vi "FlatSequenceToJson.vi"(6 "Current Path":path, 7 "Origin Path":path, 8 "error in":errorcluster, 10 "Relative Bounds":cluster{"x":i32, "y":i32, "w":i32, "h":i32}, 11 "FlatSequence in":refnum<vi>) -> (0 "error out":errorcluster, 3 "JSON":string)   [LabVIEW 2017]
doc: "Converts a flat sequence structure into a JSON"
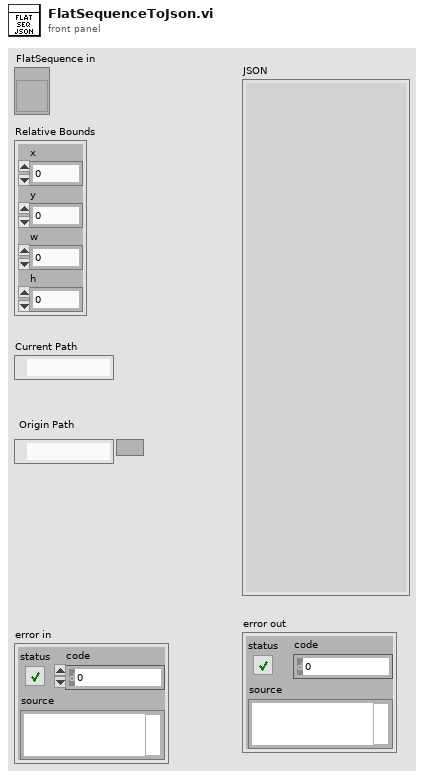
[diagram p1: front panel]
types:
  T1 = typedef "LVRectTypeDef.ctl" = cluster{"Left":i16, "Top":i16, "Right":i16, "Bottom":i16}
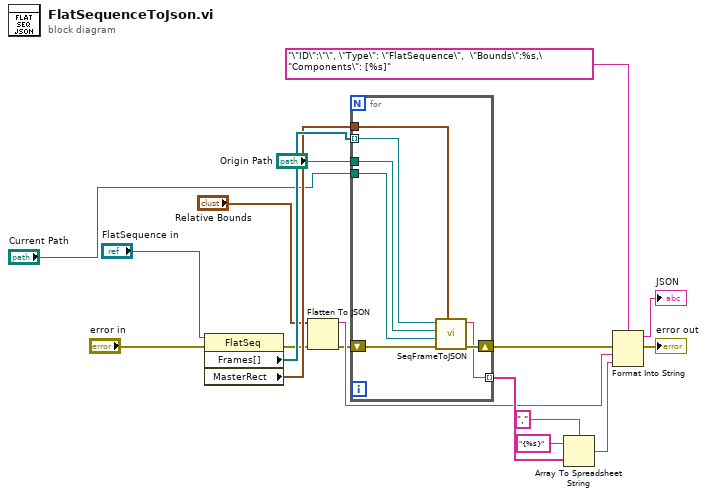
[diagram p0: block diagram]
diagram:
  n1 = property class="FlatSeq"(reference="FlatSequence in", error in="error in") -> (error out=w3:errorcluster, "Frames[]"=w17:refnum<vi>[], "MasterRect"=w12:T1)  [unwired: 1 out]
  n2 = Flatten To JSON(anything="Relative Bounds", error in (no error)=w3) -> (JSON string=w4:string, 11:w2:errorcluster)  [unwired: 1 in]
  n3 = for {
    tunnel: w17 -> [w25] mode=indexing
    shift-right: [w20] -> w15
    shift-left: w2 -> [w22]
    tunnel: w12 -> [w24]
    tunnel: "Current Path" -> [w23]
    tunnel: "Origin Path" -> [w21]
    tunnel: [w19] -> w9 mode=indexing
    n4 = call "SeqFrameToJSON.vi"("MasterRect"=w24, "error in (no error)"=w22, "created path"=w23, "Origin Path"=w21, "FlatSequenceFrame in"=w25) -> ("error out"=w20:errorcluster, "JSON"=w19:string)  [unwired: 5 in]
  }
  n5 = Array To Spreadsheet String(delimiter (Tab)=",", array=w9, 3:"{%s}" ("format string")) -> (spreadsheet string=w6:string)
  n6 = Format Into String(format string="\"ID\":\"\", \"Type\": \"FlatSequence\",  \"Bounds\":%s,\"Components\": [%s]", error in=w15, w4, w6) -> (resulting string=→"JSON":string, error out=→"error out":errorcluster)  [unwired: 1 in]
